vi "Tree Toggle Symbol.vi"(8 "error in (no error)":errorcluster, 10 "Symbol in":i32, 11 "TreeControl in":refnum<vi>) -> (0 "error out":errorcluster, 2 "Symbol out":i32, 3 "TreeControl out":refnum<vi>, 4 "Checked?":bool)   [LabVIEW 2019]
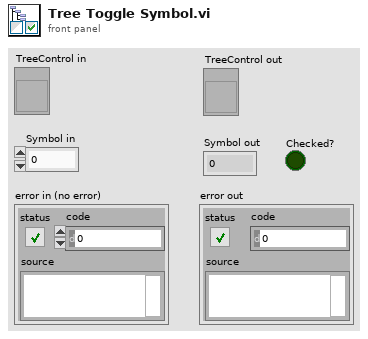
[diagram p1: front panel]
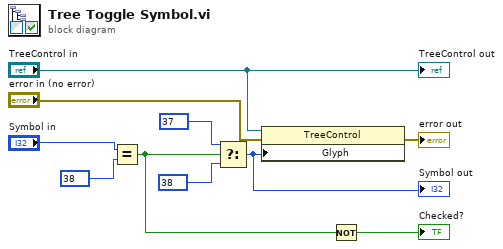
[diagram p0: block diagram]
diagram:
  n1 = Equal?(x="Symbol in", y=38) -> (x = y?=w2:bool)
  n2 = Select(t=37, s=w2, f=38) -> (s? t:f=w9:i32)
  "Symbol out" <- w9
  n3 = property class="TreeControl"(reference="TreeControl in", error in="error in (no error)", "Glyph"=w9) -> (error out=→"error out":errorcluster)  [unwired: 1 out]
  n4 = Not(x=w2) -> (.not. x?=→"Checked?":bool)
  "TreeControl out" <- "TreeControl in"
